vi "OPC Main.vi"(7 "Name of Parent Panel":string="Main.vi", 9 "New Center Coords":T1={"Horizontal"=470, "Vertical"=200}, 10 "Config":variant, 11 "Main UI Message Queue":refnum<queue>) -> ()   [LabVIEW 2018, in "OPC UA.lvlib"]
uses:
  OPC UA.lvlib
  support/Message Queue/Message Cluster.ctl
  <vilib>/Utility/miscctls.llb/LVPoint32TypeDef.ctl
  controls/UI State.ctl
  OPC Module Config.ctl
  Scale Module Folder/Measure Instrument/State Enum.ctl
  OPC Settings.ctl
  Variable Data Cluster.ctl
  <vilib>/OPCUA/controls/NodeId.ctl
  <vilib>/OPCUA/controls/OPC UA StatusCode.ctl
  <vilib>/OPCUA/controls/Subscription ID.ctl
  <vilib>/OPCUA/controls/OPC UA Client Refnum.ctl
  <vilib>/OPCUA/controls/Subscription Data Change.ctl
  <vilib>/OPCUA/controls/Data Type.ctl
  OPC Display Cluster.ctl
  support/Message Queue/Enqueue Message (Single).vi
  <vilib>/Utility/error.llb/Error Cluster From Error Code.vi
  <vilib>/ErrorRing/Error Ring.xnode
  support/Message Queue/Message Queue.lvlib
  support/Support Library.lvlib
  support/Command Log VIs/Command Logging.lvlib
  support/User Event - Stop/User Event - Stop.lvlib
  OPC Dialog.vi
  Scale Module Folder/Measure Instrument/Scale Module Engine.lvlib
  OPC UA Module Engine.lvlib
panel:
  out "Configuration.server endpoint URL":string
  out "Updating":bool
  out "ScanCode":i16
  in  "Settings Button":bool
  in  "Exit":bool
  out "Status":string
  out "Log File path":path
  out "server endpoint URL":string
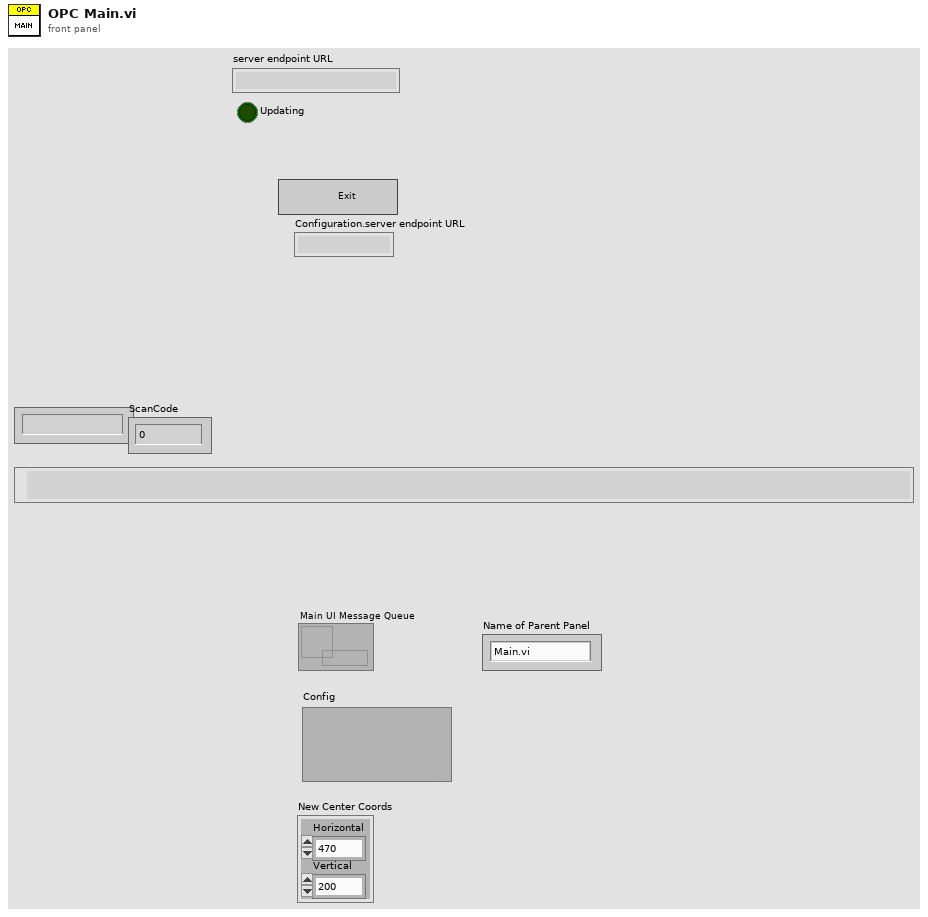
[diagram p1: front panel]
types:
  T1 = typedef "LVPoint32TypeDef.ctl" = cluster{"Horizontal":i32, "Vertical":i32}
  T2 = typedef "OPC UA.lvlib/OPC Module Config.ctl" = cluster{"State":T3, "GUID":string, "Drop Coords":T1, "Configuration":T4, "First Iteration":bool, "Data":cluster{"Object Name":string, "Variable Array":T5[]}[], "Process Name":string, "Load Count":i32, "Log Started":bool, "subscription ID out":T8, "OPC UA client refnum out":T9, "Event Registration Refnum":refnum<event-registration>, "Start Time":timestamp, "Current Time":timestamp}
  T3 = typedef "Scale Module.lvlib/Scale Module Engine.lvlib/State Enum.ctl" = enum16{"Measuring", "Idle"}
  T4 = typedef "OPC UA.lvlib/OPC Settings.ctl" = cluster{"Cycle Period":dbl, "server endpoint URL":string, "security policy":cluster{"message mode":enum16{"None", "Sign", "Sign and Encrypt"}, "security":enum16{"Basic256", "Basic128Rsa15"}}, "Trust Any Server":bool}
  T5 = typedef "OPC UA.lvlib/Variable Data Cluster.ctl" = cluster{"node ID":T6, "browse name":string, "status":T7, "timestamp":timestamp, "value ":variant}
  T6 = typedef "NodeId.ctl" = string
  T7 = typedef "OPC UA StatusCode.ctl" = u32
  T8 = typedef "Subscription ID.ctl" = u32
  T9 = typedef "OPC UA Client Refnum.ctl" = refnum<k21>
  T10 = typedef "UI State.ctl" = enum16{"Idle", "Acquiring and Logging", "Waiting for Exit", "Waiting for Exit (Acq Stopped)", "Waiting for Exit (Log Stopped)", "Waiting for Stop", "Waiting for Stop (Acq Stopped)", "Waiting for Stop (Log Stopped)"}
  T11 = typedef "OPC UA.lvlib/Message Queues.ctl" = cluster{"OPC UI":refnum<queue>, "OPC Engine":refnum<queue>, "OPC Display":refnum<queue>}
  T12 = typedef "OPC UA.lvlib/OPC Display Cluster.ctl" = cluster{"URL":string, "Cycle":i32, "Updating":bool}
  T13 = cluster{"Shift":bool, "Ctrl":bool, "Alt":bool, "Cmd":bool, "Opt":bool}
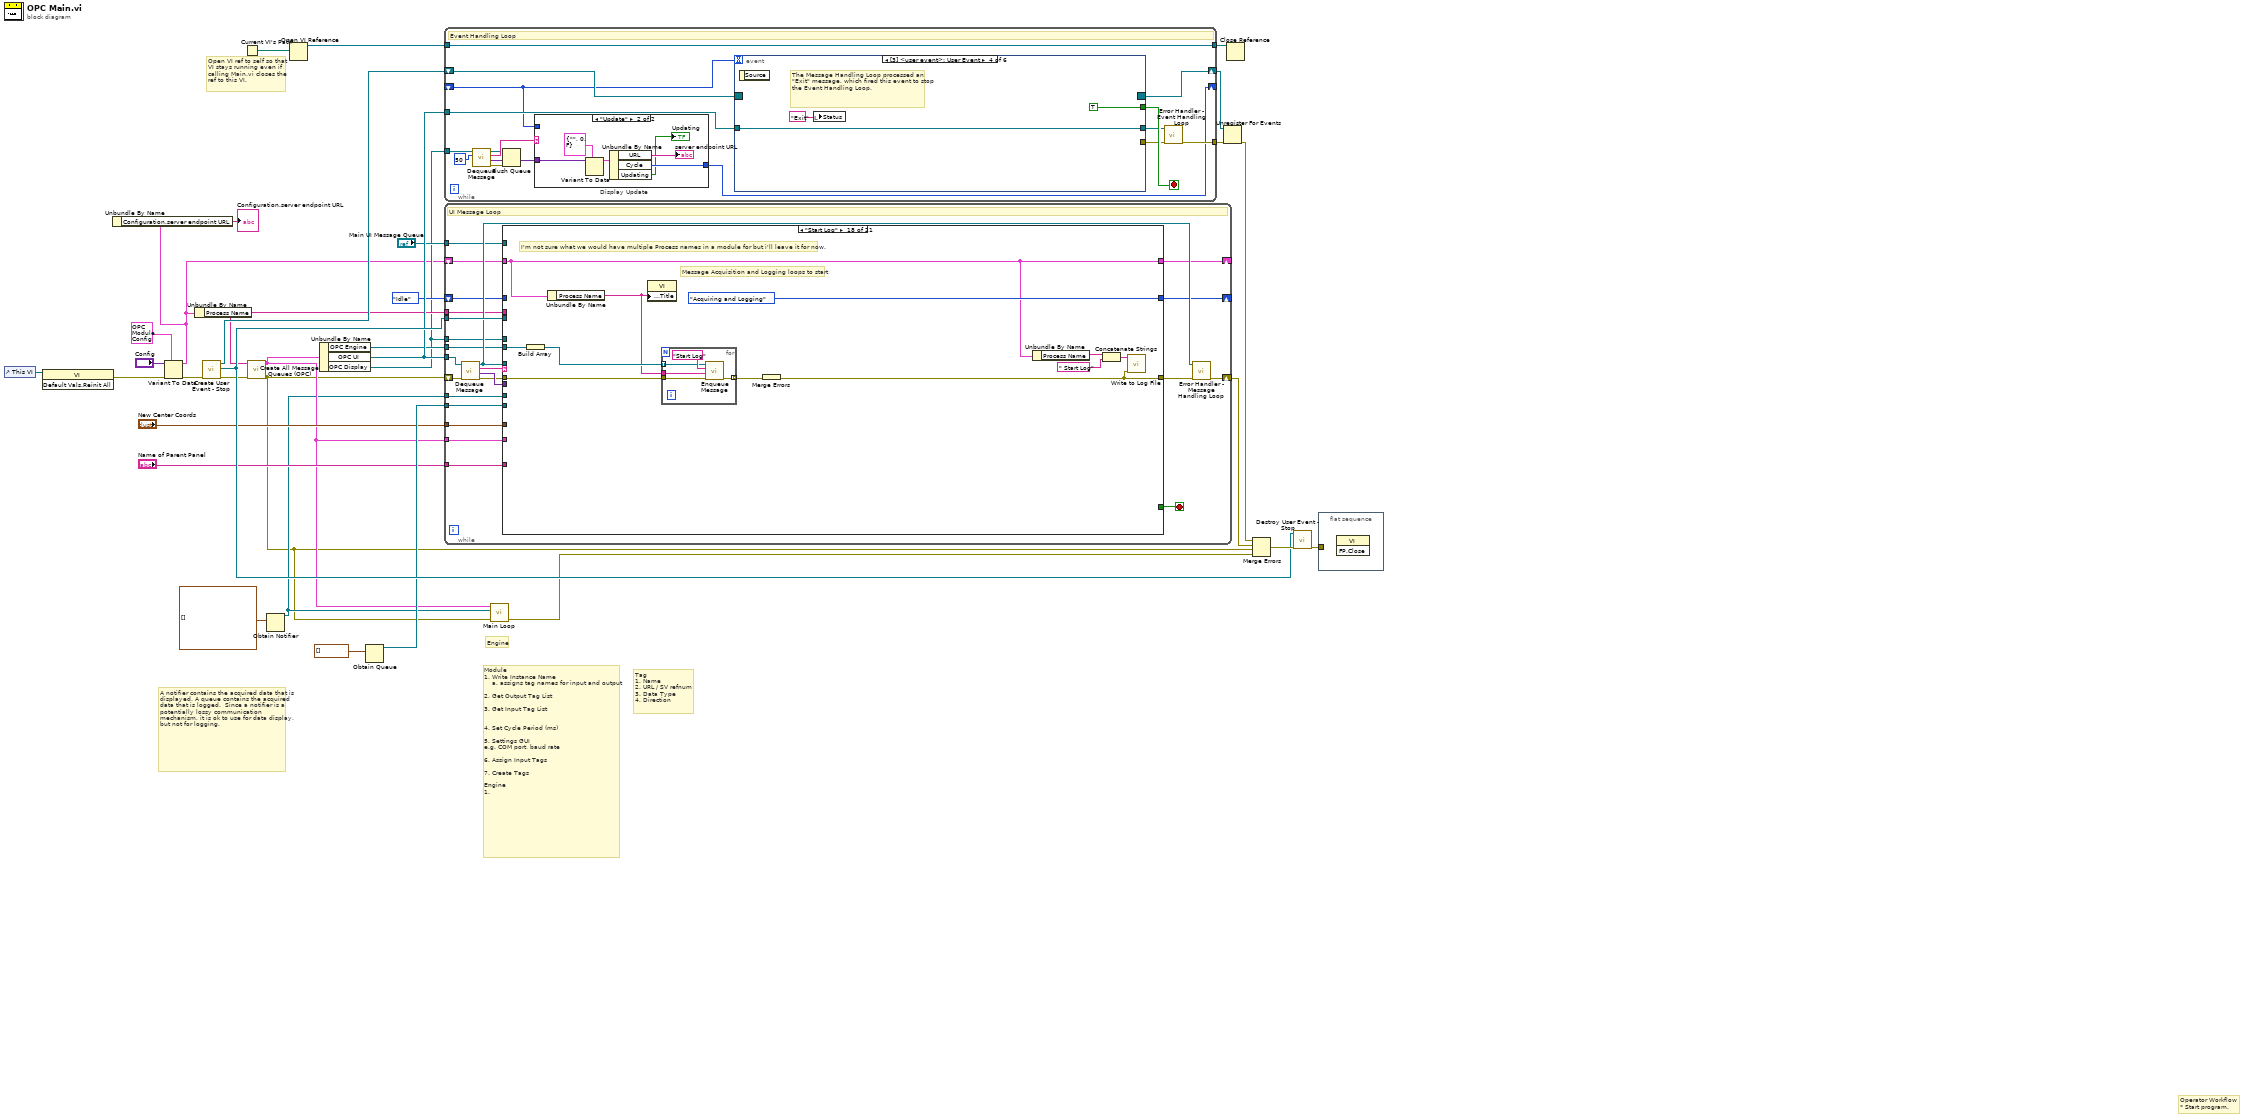
[diagram p0: block diagram]
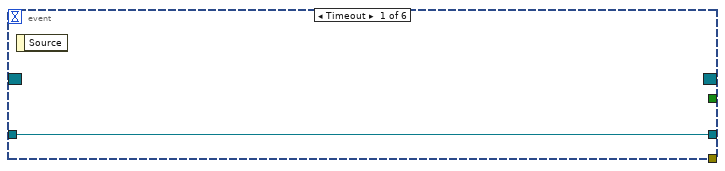
[diagram p3: hidden frame]
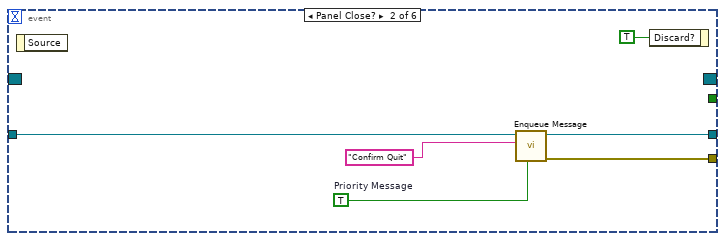
[diagram p4: hidden frame]
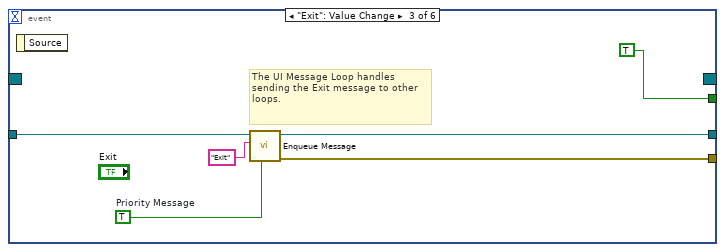
[diagram p5: hidden frame]
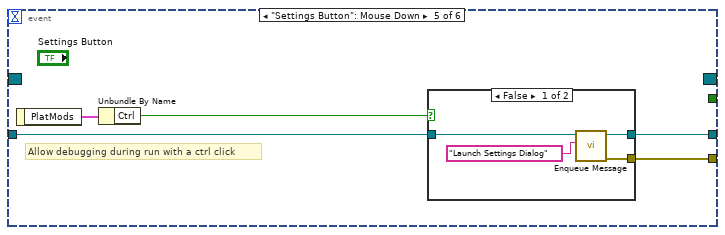
[diagram p6: hidden frame]
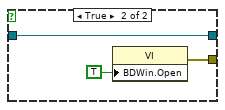
[diagram p7: hidden frame]
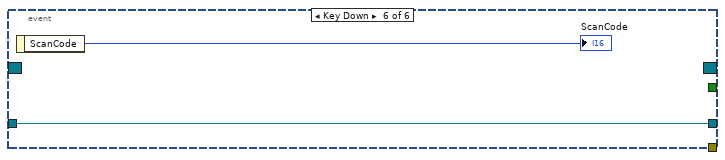
[diagram p8: hidden frame]
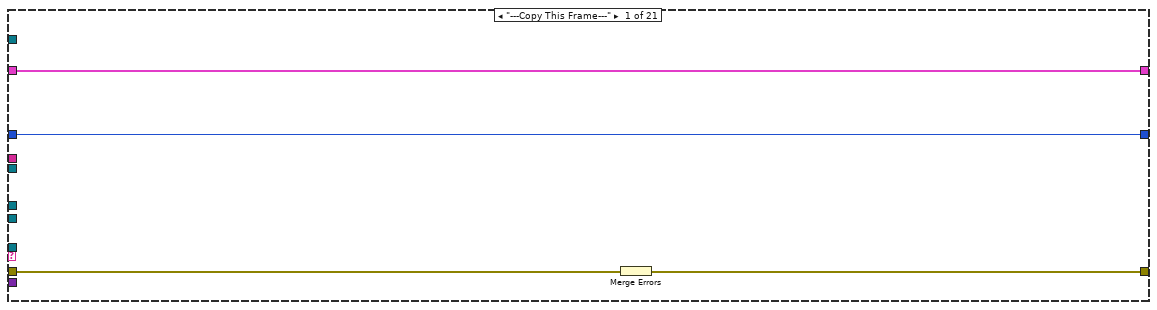
[diagram p9: hidden frame]
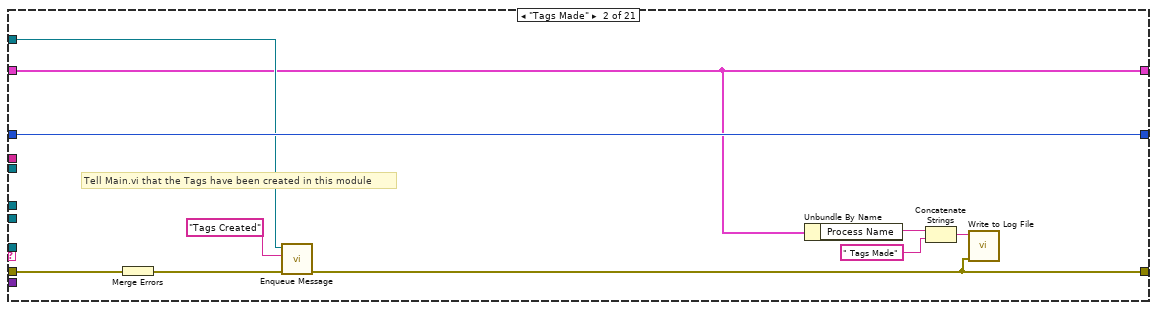
[diagram p10: hidden frame]
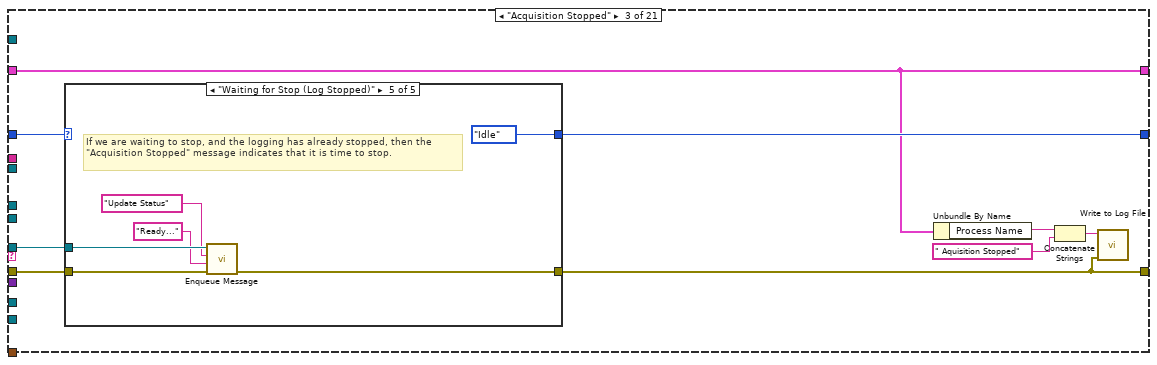
[diagram p11: hidden frame]
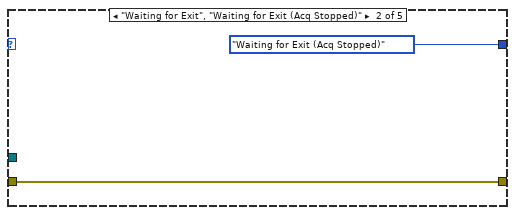
[diagram p13: hidden frame]
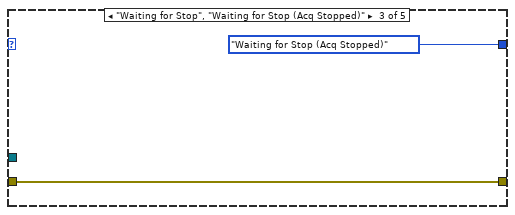
[diagram p14: hidden frame]
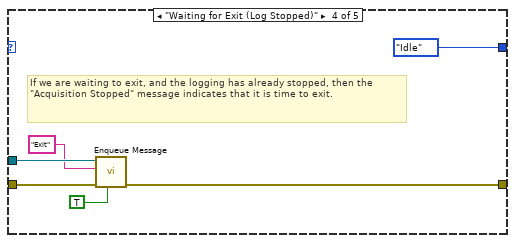
[diagram p15: hidden frame]
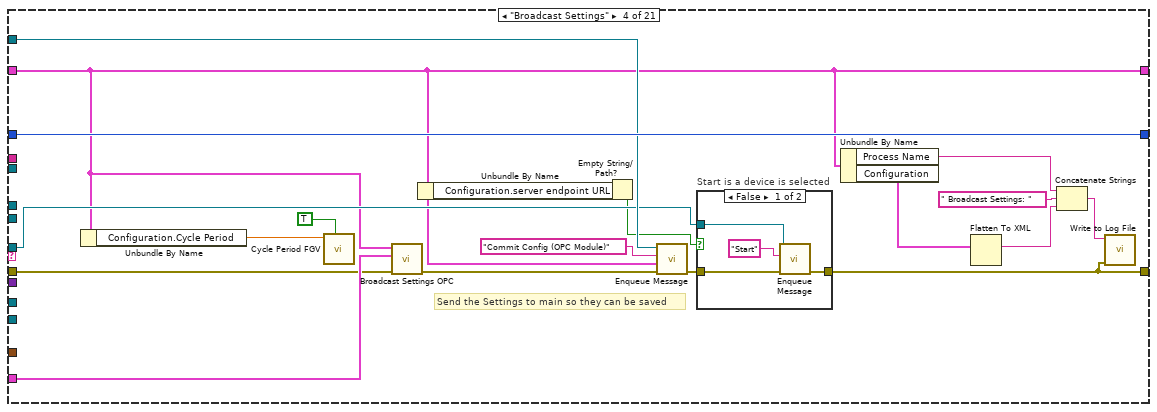
[diagram p16: hidden frame]
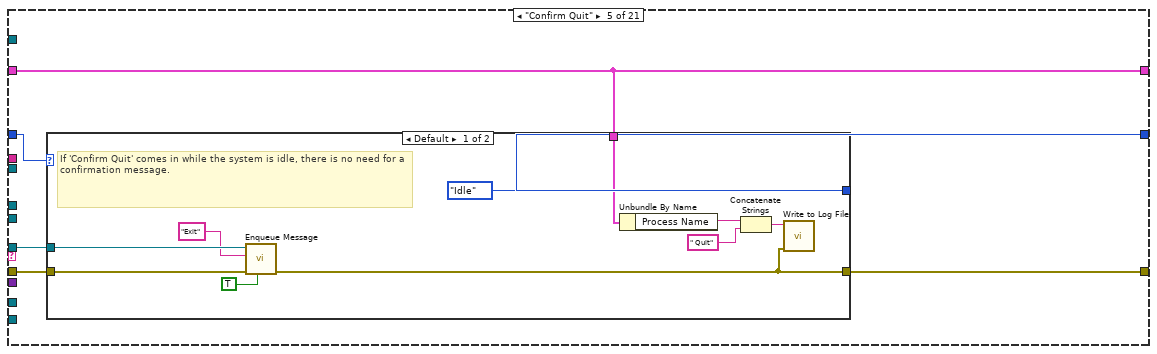
[diagram p18: hidden frame]
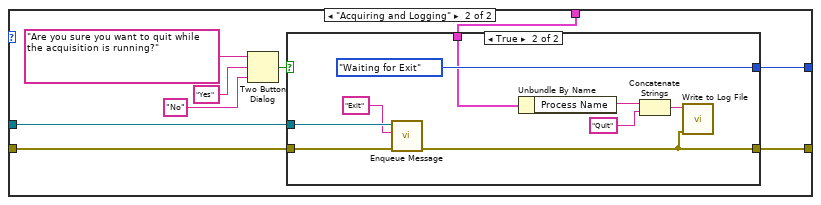
[diagram p19: hidden frame]
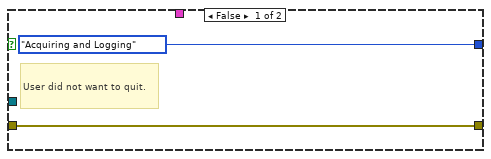
[diagram p20: hidden frame]
diagram:
  # "Open VI ref to self so that\nVI stays running even if\ncalling Main.vi closes the\nref to this VI."
  # "Engine"
  # "Operator Workflow\n* Start program."
  # "Module \n1. Write Instance Name\n    a. assigns tag names for input and output\n\n2. Get Output Tag List\n\n3. Get Input Tag List\n\n\n4. Set Cycle Period (ms)\n\n5. Settings GUI\ne.g. COM port, baud rate\n\n6. Assign Input Tags\n\n7. Create Tags\n\nEngine\n1."
  # "Tag\n1. Name\n2. URL / SV refnum\n3. Data Type\n4. Direction"
  # "A notifier contains the acquired data that is displayed. A queue contains the acquired data that is logged.  Since a notifier is a potentially lossy communication mechanism, it is ok to use for data display, but not for logging."
  n1 = control-ref of="This VI"() -> (w3:refnum<vi>)
  n2 = invoke class="VI" method="Default Vals.Reinit All"(reference=w3) -> (error out=w13:errorcluster)  [unwired: 2 in, 2 out]
  n3 = Variant To Data(error in=w13, type=T2 {"State"=enum."Idle", "GUID"="", "Drop Coords"={"Horizontal"=0, "Vertical"=0}, "Configuration"={"Cycle Period"=500.0, "server endpoint URL"="", "security policy"={"message mode"=enum."Sign", "security"=enum."Basic256"}, "Trust Any Server"=FALSE}, "First Iteration"=FALSE, "Data"=[], "Process Name"="", "Load Count"=0, "Log Started"=FALSE, "subscription ID out"=0, "OPC UA client refnum out"="", "Event Registration Refnum"=refnum, "Start Time"=timestamp(0 s since 1904-01-01), "Current Time"=timestamp(0 s since 1904-01-01)} ("OPC Module Config"), Variant="Config") -> (data=w2:T2, error out=w18:errorcluster)
  n4 = Unbundle By Name(w2) -> ("Configuration.server endpoint URL"=→"Configuration.server endpoint URL":string)
  n5 = Unbundle By Name(w2) -> ("Process Name"=w12:string)
  n6 = call "Create User Event - Stop.vi"("error in (no error)"=w18) -> ("error out"=w11:errorcluster, "User Event - Stop"=w30:refnum<user-event>, "Stop Event Registration Refnum"=w31:refnum<event-registration>)  [unwired: 8 in]
  n7 = Current VI's Path() -> (path=w19:path)
  n8 = call "Create All Message Queues (OPC).vi"("error in (no error)"=w11, "Process Name"=w12) -> ("error out"=w8:errorcluster, "Message Queues"=w10:T11)  [unwired: 8 in]
  n9 = Obtain Notifier(notification data type=waveform(dbl)[] []) -> (notifier out=w9:refnum<notifier>)  [unwired: 3 in, 2 out]
  n10 = Open VI Reference(vi path=w19) -> (vi reference=w20:refnum<vi>)  [unwired: 5 in, 1 out]
  n11 = Unbundle By Name(w10) -> ("OPC Engine"=w23:refnum<queue>, "OPC UI"=w27:refnum<queue>, "OPC Display"=w4:refnum<queue>)
  n12 = Obtain Queue(element data type=waveform(dbl)[] []) -> (queue out=w22:refnum<queue>)  [unwired: 4 in, 2 out]
  n13 = while {
    tunnel: w27 -> [w52]
    tunnel: w30 -> [w56]
    shift-right: [w48] -> w34
    shift-left: w8 -> [w55]
    shift-right: [w39] -> _
    shift-left: w2 -> [w41]
    tunnel: w9 -> [w51]
    tunnel: w22 -> [w50]
    shift-right: [w45] -> _
    shift-left: UI_State."Idle" ("UI State") -> [w46]
    tunnel: w23 -> [w44]
    tunnel: w10 -> [w43]
    tunnel: "Main UI Message Queue" -> [w40]
    tunnel: w12 -> [w38]
    tunnel: "New Center Coords" -> [w37]
    tunnel: "Name of Parent Panel" -> [w36]
    tunnel: w4 -> [w35]
    stop <- w57 stop-if-true
    # "UI Message Loop"
    n14 = call "Dequeue Message.vi"("error in (no error)"=w55, "Message Queue"=w52) -> ("error out"=w42:errorcluster, "Message Data"=w53:variant, "Message"=w54:string, "dup Message Queue"=w47:refnum<queue>)  [unwired: 6 in]
    n15 = case "Message Cases" shown="\"Start Log\"" w54 {
      selector: w54 -> [_ _ _ _ _ _ _ _ _ _ _ _ _ _ _ _ _ _ _ _ w396]
      tunnel: w47 -> [_ _ w77 w112 w127 _ w177 w191 w213 _ w256 w273 w289 w312 w320 w338 _ _ w385 _ _]
      tunnel: w42 -> [w61 w71 w78 w100 w126 w161 w172 w195 w212 w238 w252 w265 w290 w313 w319 w337 w344 w361 w380 w394 _]
      tunnel: [w60 w62 w73 w107 w125 w162 w167 w182 w197 w238 w241 w269 w285 w311 w318 w333 w349 w356 w372 w395 w398] -> w49
      tunnel: [_ _ _ _ _ _ _ _ TRUE _ _ _ _ _ _ _ _ _ _ _ _] -> w57
      tunnel: w53 -> [_ _ _ _ _ w164 _ w194 w202 _ _ _ _ _ _ _ _ _ _ w393 _]
      tunnel: w56 -> [_ _ _ _ _ _ _ _ w223 _ _ _ _ _ _ _ _ _ _ _ _]
      tunnel: w41 -> [w58 w63 w72 w106 w123 w159 w166 w181 w196 w235 w244 w268 w284 w317 w324 w332 w342 w355 w371 w388 w397]
      tunnel: w51 -> [_ _ _ _ _ _ _ _ w221 _ _ _ _ _ _ _ _ _ _ _ _]
      tunnel: w50 -> [_ _ _ _ _ _ _ _ w217 _ _ _ _ _ _ _ _ _ _ _ _]
      tunnel: w46 -> [w59 w70 w80 w117 w128 w160 w173 w186 w210 _ _ w277 w292 w316 w323 _ _ _ w381 w389 w402]
      tunnel: [w59 w70 w79 w117 w124 w160 w174 w186 w209 UI_State."Idle" ("UI State") UI_State."Idle" ("UI State") w277 w291 w316 w323 UI_State."Acquiring and Logging" ("UI State") UI_State."Acquiring and Logging" ("UI State") UI_State."Acquiring and Logging" ("UI State") w382 w389 w402] -> w45
      tunnel: w44 -> [_ _ _ _ _ _ _ _ w216 _ _ _ _ _ _ _ w347 w364 w379 _ _]
      tunnel: w43 -> [_ _ _ w101 _ _ _ _ _ _ _ _ _ _ _ _ _ _ _ _ _]
      tunnel: w40 -> [_ w67 _ w113 _ _ _ _ w201 _ _ w274 _ _ _ _ _ _ _ _ _]
      tunnel: [w58 w63 w72 w106 w123 w159 w166 w181 w196 w235 w244 w263 w284 w317 w324 w332 w342 w355 w371 w388 w397] -> w39
      tunnel: w38 -> [_ _ _ _ _ _ _ _ _ _ w250 _ _ _ _ _ _ _ _ _ _]
      tunnel: w37 -> [_ _ _ _ _ _ _ _ _ _ w249 _ _ _ _ _ _ _ _ _ _]
      tunnel: w36 -> [_ _ _ _ _ _ _ _ _ _ w248 _ _ _ _ _ _ _ _ _ _]
      tunnel: w35 -> [_ _ _ _ _ _ _ _ _ _ w243 _ _ _ _ _ _ _ _ _ _]
      frame "---Copy This Frame---" {
        # "Duplicate this frame when creating new messages.  Change this comment in the duplicated frame to describe this message."
        n16 = Merge Errors(w61) -> (w60:errorcluster)
      }
      frame "Tags Made" {
        # "Tell Main.vi that the Tags have been created in this module"
        # "Duplicate this frame when creating new messages.  Change this comment in the duplicated frame to describe this message."
        n17 = Merge Errors(w71) -> (w68:errorcluster)
        n18 = call-poly "Enqueue Message.vi"("error in (no error)"=w68, "Message"="Tags Created", "Message Queue"=w67) -> ("error out"=w62:errorcluster)  [unwired: 7 in, 1 out]
        n19 = Unbundle By Name(w63) -> ("Process Name"=w66:string)
        n20 = Concatenate Strings(w66, " Tags Made" ("text")) -> (w64:string)
        n21 = call "Write to Log File.vi"("error in"=w62, "text"=w64) -> ()  [unwired: 9 in, 1 out]
      }
      frame "Acquisition Stopped" {
        # "Logic for determining what action to take when the acquisition has stopped."
        n22 = case shown="\"Waiting for Stop (Log Stopped)\"" w80 {
          selector: w80 -> [w82 _ _ _ _]
          tunnel: [w82 UI_State."Waiting for Exit (Acq Stopped)" ("UI State") UI_State."Waiting for Stop (Acq Stopped)" ("UI State") UI_State."Idle" ("UI State") UI_State."Idle" ("UI State")] -> w79
          tunnel: w78 -> [w81 w83 w85 w91 w97]
          tunnel: [w81 w83 w85 w90 w96] -> w73
          tunnel: w77 -> [_ _ _ w89 w95]
          frame Default {
          }
          frame "Waiting for Exit", "Waiting for Exit (Acq Stopped)" {
          }
          frame "Waiting for Stop", "Waiting for Stop (Acq Stopped)" {
          }
          frame "Waiting for Exit (Log Stopped)" {
            # "If we are waiting to exit, and the logging has already stopped, then the \"Acquisition Stopped\" message indicates that it is time to exit."
            n23 = call-poly "Enqueue Message.vi"("Priority Message? (F)"=TRUE, "error in (no error)"=w91, "Message"="Exit", "Message Queue"=w89) -> ("error out"=w90:errorcluster)  [unwired: 6 in, 1 out]
          }
          frame "Waiting for Stop (Log Stopped)" {
            # "If we are waiting to stop, and the logging has already stopped, then the \"Acquisition Stopped\" message indicates that it is time to stop."
            n24 = call-poly "Enqueue Message.vi"("error in (no error)"=w97, "Message Data"="Ready..." ("Message"), "Message"="Update Status", "Message Queue"=w95) -> ("error out"=w96:errorcluster)  [unwired: 6 in, 1 out]
          }
        }
        n25 = Unbundle By Name(w72) -> ("Process Name"=w76:string)
        n26 = Concatenate Strings(w76, " Aquisition Stopped" ("text")) -> (w74:string)
        n27 = call "Write to Log File.vi"("error in"=w73, "text"=w74) -> ()  [unwired: 9 in, 1 out]
      }
      frame "Broadcast Settings" {
        # "Send the Settings to main so they can be saved"
        # "Send the 'Update Settings' message to the Logging and Acquisition message loops."
        n28 = Unbundle By Name(w106) -> ("Configuration.Cycle Period"=w115:dbl)
        n29 = call "Cycle Period FGV.vi"("Write"=TRUE, "Cycle Period In (ms)"=w115) -> ()  [unwired: 8 in, 2 out]
        n30 = call "Broadcast Settings OPC.vi"("error in (no error)"=w100, "Message Queues"=w101, "OPC Module Config"=w106) -> ("error out"=w99:errorcluster)  [unwired: 8 in]
        n31 = Unbundle By Name(w106) -> ("Configuration.server endpoint URL"=w103:string)
        n32 = Empty String/Path?(string/path=w103) -> (empty?=w102:bool)
        n33 = call-poly "Enqueue Message.vi"("error in (no error)"=w99, "Message Data"=w106, "Message"="Commit Config (OPC Module)", "Message Queue"=w113) -> ("error out"=w111:errorcluster)  [unwired: 6 in, 1 out]
        n34 = case "Start is a device is selected" shown="False" w102 {
          tunnel: w112 -> [w120 _]
          tunnel: w111 -> [w119 w122]
          tunnel: [w118 w122] -> w107
          frame False {
            n35 = call-poly "Enqueue Message.vi"("error in (no error)"=w119, "Message"="Start", "Message Queue"=w120) -> ("error out"=w118:errorcluster)  [unwired: 7 in, 1 out]
          }
          frame True {
          }
        }
        n36 = Unbundle By Name(w106) -> ("Process Name"=w110:string, "Configuration"=w105:T4)
        n37 = Flatten To XML(anything=w105) -> (xml string=w104:string)
        n38 = Concatenate Strings(w110, " Broadcast Settings: " ("text"), w104) -> (w108:string)
        n39 = call "Write to Log File.vi"("error in"=w107, "text"=w108) -> ()  [unwired: 9 in, 1 out]
      }
      frame "Confirm Quit" {
        # "Confirm Quit - Message that can confirm whether or not the user wants to exit the application."
        n40 = case shown="Default" w128 {
          tunnel: w127 -> [w137 w144]
          tunnel: w126 -> [w136 w142]
          tunnel: [w130 w141] -> w125
          tunnel: [UI_State."Idle" ("UI State") w140] -> w124
          tunnel: w123 -> [w129 w139]
          frame Default {
            # "If 'Confirm Quit' comes in while the system is idle, there is no need for a confirmation message."
            n41 = call-poly "Enqueue Message.vi"("Priority Message? (F)"=TRUE, "error in (no error)"=w136, "Message"="Exit", "Message Queue"=w137) -> ("error out"=w130:errorcluster)  [unwired: 6 in, 1 out]
            n42 = Unbundle By Name(w129) -> ("Process Name"=w133:string)
            n43 = Concatenate Strings(w133, " Quit" ("text")) -> (w131:string)
            n44 = call "Write to Log File.vi"("error in"=w130, "text"=w131) -> ()  [unwired: 9 in, 1 out]
          }
          frame "Acquiring and Logging" {
            n45 = Two Button Dialog(message="Are you sure you want to quit while the acquisition is running?" ("Confirm Quit Message"), 1:"No" ("No"), 2:"Yes" ("Yes")) -> (T button?=w143:bool)
            n46 = case shown="True" w143 {
              tunnel: w144 -> [_ w158]
              tunnel: w142 -> [w148 w157]
              tunnel: [w148 w151] -> w141
              tunnel: [UI_State."Acquiring and Logging" ("UI State") UI_State."Waiting for Exit" ("UI State")] -> w140
              tunnel: w139 -> [_ w150]
              frame False {
                # "User did not want to quit."
              }
              frame True {
                n47 = call-poly "Enqueue Message.vi"("error in (no error)"=w157, "Message"="Exit", "Message Queue"=w158) -> ("error out"=w151:errorcluster)  [unwired: 7 in, 1 out]
                n48 = Unbundle By Name(w150) -> ("Process Name"=w154:string)
                n49 = Concatenate Strings(w154, "Quit" ("text")) -> (w152:string)
                n50 = call "Write to Log File.vi"("error in"=w151, "text"=w152) -> ()  [unwired: 9 in, 1 out]
              }
            }
          }
        }
      }
      frame "Display Log File Path" {
        n51 = Variant To Data(error in=w161, type=path "", Variant=w164) -> (data=→"Log File path":path, error out=w162:errorcluster)
      }
      frame "E-Stop" {
        # "E-Stop has no effect on the scale"
        # "Message Acquisition and Logging loops to stop"
        # "Stop the pumps."
        n52 = call-poly "Enqueue Message.vi"("error in (no error)"=w172, "Message Data"="Ready..." ("Ready..."), "Message"="Update Status", "Message Queue"=w177) -> ("error out"=w171:errorcluster)  [unwired: 6 in, 1 out]
        n53 = case shown="\"Waiting for Exit\"" w173 {
          selector: w173 -> [_ w179]
          tunnel: [UI_State."Waiting for Stop" ("UI State") w179] -> w174
          frame Default {
          }
          frame "Waiting for Exit" {
          }
        }
        n54 = Merge Errors(w171) -> (w167:errorcluster)
        n55 = Unbundle By Name(w166) -> ("Process Name"=w170:string)
        n56 = Concatenate Strings(w170, " E-STOP" ("text")) -> (w168:string)
        n57 = call "Write to Log File.vi"("error in"=w167, "text"=w168) -> ()  [unwired: 9 in, 1 out]
      }
      frame "Error" {
        # "Error - Check the error message data and respond accordingly. This message is sent by the \"Error Handler\" VIs at the end of each loop in this application."
        n58 = Variant To Data(error in=w195, type=errorcluster {"status"=FALSE, "code"=0, "source"=""} ("error out"), Variant=w194) -> (data=w192:errorcluster, error out=w188:errorcluster)
        n59 = call <vilib>:"General Error Handler.vi"("error in (no error)"=w192) -> ("message"=w180:string)  [unwired: 10 in, 4 out]
        n60 = call-poly "Enqueue Message.vi"("Priority Message? (F)"=TRUE, "Message"="Exit", "Message Queue"=w191) -> ("error out"=w187:errorcluster)  [unwired: 7 in, 1 out]
        n61 = Merge Errors(w187, w188) -> (w182:errorcluster)
        n62 = Unbundle By Name(w181) -> ("Process Name"=w185:string)
        n63 = Concatenate Strings(w185, " Error: " ("text"), w180) -> (w183:string)
        n64 = call "Write to Log File.vi"("error in"=w182, "text"=w183) -> ()  [unwired: 9 in, 1 out]
      }
      frame "Exit" {
        w205 = TRUE  # Delete Module?
        # "Don't check the error outs. The acquisition and logging queues may have already been released."
        # "Close references owned by the Main VI."
        # "Stop the VI"
        # "Exit - Fire the User Event to stop the Event Handling Loop.  Also send Exit messages to the Acquisition and Logging loops."
        n65 = call "Fire User Event - Stop.vi"("User Event - Stop"=w223) -> ("error out"=w222:errorcluster)  [unwired: 10 in]
        n66 = Build Array(w216) -> (w215:refnum<queue>[])
        n67 = for {
          tunnel: w215 -> [w232] mode=indexing
          n68 = call-poly "Enqueue Message.vi"("Message"="Stop", "Message Queue"=w232) -> ("dup Message Queue"=w233:refnum<queue>)  [unwired: 8 in, 1 out]
          n69 = call-poly "Enqueue Message.vi"("Message"="Exit", "Message Queue"=w233) -> ()  [unwired: 8 in, 2 out]
        }
        n70 = Variant To Data(type=w205, Variant=w202) -> (data=w204:bool, error out=w206:errorcluster)  [unwired: 1 in]
        n71 = call-poly "Enqueue Message.vi"("error in (no error)"=w212, "Message Data"="Ready..." ("Ready..."), "Message"="Update Status", "Message Queue"=w213) -> ("error out"=w211:errorcluster, "dup Message Queue"=w208:refnum<queue>)  [unwired: 6 in]
        n72 = Select(t=w205, s=w206, f=w204) -> (s? t:f=w203:bool)
        n73 = case "Don't enqueue Delete Module if opening campaign because it\nwill already have been deleted and new config loaded and we create\na race condition." shown="True" w203 {
          tunnel: w201 -> [_ w227]
          tunnel: w196 -> [_ w226]
          frame False {
          }
          frame True {
            n74 = Unbundle By Name(w226) -> ("GUID"=w225:string)
            n75 = call-poly "Enqueue Message.vi"("Message Data"=w225, "Message"="Delete Module", "Message Queue"=w227) -> ()  [unwired: 7 in, 2 out]
          }
        }
        n76 = Release Queue(queue=w208, error in (no error)=w211) -> (error out=w220:errorcluster)  [unwired: 1 in, 2 out]
        n77 = Release Notifier(notifier=w221, error in (no error)=w220) -> (error out=w219:errorcluster)  [unwired: 1 in, 2 out]
        n78 = Release Queue(queue=w217, error in (no error)=w219) -> (error out=w218:errorcluster)  [unwired: 1 in, 2 out]
        n79 = Merge Errors(w222, w218) -> (w197:errorcluster)
        n80 = case shown="Default" w210 {
          selector: w210 -> [_ w230]
          tunnel: [UI_State."Waiting for Stop" ("UI State") w230] -> w209
          frame Default {
          }
          frame "Waiting for Exit" {
          }
        }
        n81 = Unbundle By Name(w196) -> ("Process Name"=w200:string)
        n82 = Concatenate Strings(w200, " Exit" ("text")) -> (w198:string)
        n83 = call "Write to Log File.vi"("error in"=w197, "text"=w198) -> ()  [unwired: 9 in, 1 out]
      }
      frame "Init UI Refs" {
        # "Init UI Refs - Store control references for UI controls.  Also enable/disable controls appropriately."
        n84 = property class="VI"("Front Panel.Closeable"=TRUE ("Front Panel Window:Closeable")) -> ()  [unwired: 2 in, 2 out]
      }
      frame "Initialize" {
        # "Initialize - Get configuration settings, then message the UI to initialize, and broadcast the settings to the other message loops."
        n85 = call-poly "Enqueue Message.vi"("error in (no error)"=w252, "Message"="Init UI Refs", "Message Queue"=w256) -> ("error out"=w254:errorcluster, "dup Message Queue"=w255:refnum<queue>)  [unwired: 7 in]
        n86 = property class="VI" props=["FP.State"]() -> (reference out=w251:refnum<vi>)  [unwired: 2 in, 2 out]
        n87 = call "Make Child and Move.vi"("Process Name"=w250, "Name of Parent Panel"=w248, "New Center Coords"=w249, "VI in"=w251) -> ()  [unwired: 8 in]
        n88 = call-poly "Enqueue Message.vi"("error in (no error)"=w254, "Message"="Broadcast Settings", "Message Queue"=w255) -> ("error out"=w262:errorcluster, "dup Message Queue"=w261:refnum<queue>)  [unwired: 7 in]
        n89 = call-poly "Enqueue Message.vi"("error in (no error)"=w262, "Message Data"="Ready..." ("Ready..."), "Message"="Update Status", "Message Queue"=w261) -> ("error out"=w242:errorcluster)  [unwired: 6 in, 1 out]
        n90 = call-poly "Enqueue Message.vi"("error in (no error)"=w242, "Message Data"=T12 {"URL"="", "Cycle"=0, "Updating"=FALSE} ("OPC Display Cluster"), "Message"="Update", "Message Queue"=w243) -> ("error out"=w241:errorcluster)  [unwired: 6 in, 1 out]
        n91 = Unbundle By Name(w244) -> ("Process Name"=w247:string)
        n92 = Concatenate Strings(w247, " Initialize" ("text")) -> (w245:string)
        n93 = call "Write to Log File.vi"("error in"=w241, "text"=w245) -> ()  [unwired: 9 in, 1 out]
      }
      frame "Launch Settings Dialog" {
        # "Launch the Settings Dialog when the user clicks the 'Settings' button."
        n94 = Unbundle By Name(w268) -> ("Load Count"=w275:i32)
        n95 = Increment(x=w275) -> (x+1=w276:i32)
        n96 = Bundle By Name(cluster=w268, "Load Count"=w276) -> (w264:T2)
        n97 = call-by-ref "?"("error in (no error)"=w265, "OPC Module Config In"=w264) -> ("error out"=w266:errorcluster, "Cancelled?"=w267:bool, "OPC Module Config Out"=w263:T2)  [unwired: 8 in, 3 out]
        n98 = case shown="False" w267 {
          tunnel: w266 -> [w280 w283]
          tunnel: [w279 w283] -> w269
          tunnel: w274 -> [_ _]
          tunnel: w273 -> [w282 _]
          tunnel: w263 -> [w278 _]
          frame False {
            n99 = call-poly "Enqueue Message.vi"("error in (no error)"=w280, "Message Data"=w278, "Message"="Broadcast Settings", "Message Queue"=w282) -> ("error out"=w279:errorcluster)  [unwired: 6 in, 1 out]
          }
          frame True {
          }
        }
        n100 = Unbundle By Name(w263) -> ("Process Name"=w272:string)
        n101 = Concatenate Strings(w272, " Setting Dialog Launched" ("text")) -> (w270:string)
        n102 = call "Write to Log File.vi"("error in"=w269, "text"=w270) -> ()  [unwired: 9 in, 1 out]
      }
      frame "Logging Stopped" {
        # "Logic for determining what action to take when the logging has stopped."
        n103 = case shown="\"Waiting for Exit (Acq Stopped)\"" w292 {
          selector: w292 -> [w294 _ _ _ _]
          tunnel: [w294 UI_State."Waiting for Exit (Log Stopped)" ("UI State") UI_State."Waiting for Stop (Log Stopped)" ("UI State") UI_State."Idle" ("UI State") UI_State."Idle" ("UI State")] -> w291
          tunnel: w290 -> [w293 w295 w297 w303 w309]
          tunnel: [w293 w295 w297 w302 w308] -> w285
          tunnel: w289 -> [_ _ _ w301 w307]
          frame Default {
          }
          frame "Waiting for Exit", "Waiting for Exit (Log Stopped)" {
          }
          frame "Waiting for Stop", "Waiting for Stop (Log Stopped)" {
          }
          frame "Waiting for Exit (Acq Stopped)" {
            # "If we are waiting to exit, and the acquisition has already stopped, then the \"Logging Stopped\" message indicates that it is time to exit."
            n104 = call-poly "Enqueue Message.vi"("Priority Message? (F)"=TRUE, "error in (no error)"=w303, "Message"="Exit", "Message Queue"=w301) -> ("error out"=w302:errorcluster)  [unwired: 6 in, 1 out]
          }
          frame "Waiting for Stop (Acq Stopped)" {
            # "If we are waiting to stop, and the acquisition has already stopped, then the \"Logging Stopped\" message indicates that it is time to stop."
            n105 = call-poly "Enqueue Message.vi"("error in (no error)"=w309, "Message Data"="Ready..." ("Message"), "Message"="Update Status", "Message Queue"=w307) -> ("error out"=w308:errorcluster)  [unwired: 6 in, 1 out]
          }
        }
        n106 = Unbundle By Name(w284) -> ("Process Name"=w288:string)
        n107 = Concatenate Strings(w288, " Logging Stopped" ("text")) -> (w286:string)
        n108 = call "Write to Log File.vi"("error in"=w285, "text"=w286) -> ()  [unwired: 9 in, 1 out]
      }
      frame "Send to Sequencer" {
        n109 = local read "Status"() -> (w314:string)
        n110 = call-poly "Enqueue Message.vi"("error in (no error)"=w313, "Message Data"=w314, "Message"="Sent to Sequence", "Message Queue"=w312) -> ("error out"=w311:errorcluster)  [unwired: 6 in, 1 out]
      }
      frame "Sent to Sequence" {
        n111 = local read "Status"() -> (w321:string)
        n112 = flat-sequence {
          tunnel: w319 -> [w329]
          tunnel: w320 -> [w327]
          tunnel: [w328] -> w322
          tunnel: w321 -> [w325]
          tunnel: [w331] -> w318
          tunnel: w322 -> [w331]
          frame #0 {
            n113 = call-poly "Enqueue Message.vi"("error in (no error)"=w329, "Message Data"=w325, "Message"="Sent to Sequence", "Message Queue"=w327) -> ("error out"=w328:errorcluster)  [unwired: 6 in, 1 out]
          }
          frame #1 {
            n114 = Wait (ms)(milliseconds to wait=u32 50) -> ()  [unwired: 1 out]
          }
        }
      }
      frame "Start" {
        # "Message Acquisition and Logging loops to start"
        # "Start - Enable/Disable buttons appropriately for an acquisition that has started, and update status display."
        n115 = call-poly "Enqueue Message.vi"("error in (no error)"=w337, "Message"="Start Loops", "Message Queue"=w338) -> ("error out"=w339:errorcluster)  [unwired: 7 in, 1 out]
        n116 = Merge Errors(w339) -> (w333:errorcluster)
        n117 = Unbundle By Name(w332) -> ("Process Name"=w336:string)
        n118 = Concatenate Strings(w336, " Start" ("text")) -> (w334:string)
        n119 = call "Write to Log File.vi"("error in"=w333, "text"=w334) -> ()  [unwired: 9 in, 1 out]
      }
      frame "Start Loops" {
        # "I'm not sure what we would have multiple Process names in a module for but i'll leave it for now."
        # "Message Acquisition and Logging loops to start"
        # "Start - Enable/Disable buttons appropriately for an acquisition that has started, and update status display."
        n120 = Build Array(w347) -> (w345:refnum<queue>[])
        n121 = Unbundle By Name(w342) -> ("Process Name"=w343:string)
        n122 = property class="VI"("Front Panel.Title"=w343) -> ()  [unwired: 2 in, 2 out]
        n123 = for {
          tunnel: w344 -> [w353]
          tunnel: [w352] -> w346 mode=indexing
          tunnel: w345 -> [w351] mode=indexing
          tunnel: w343 -> [w350]
          n124 = call-poly "Enqueue Message.vi"("error in (no error)"=w353, "Message Data"=w350, "Message"="Start", "Message Queue"=w351) -> ("error out"=w352:errorcluster)  [unwired: 6 in, 1 out]
        }
        n125 = Merge Errors(w346) -> (w349:errorcluster)
      }
      frame "Start Log" {
        # "I'm not sure what we would have multiple Process names in a module for but i'll leave it for now."
        # "Message Acquisition and Logging loops to start"
        # "Start - Enable/Disable buttons appropriately for an acquisition that has started, and update status display."
        n126 = Build Array(w364) -> (w362:refnum<queue>[])
        n127 = Unbundle By Name(w355) -> ("Process Name"=w360:string)
        n128 = property class="VI"("Front Panel.Title"=w360) -> ()  [unwired: 2 in, 2 out]
        n129 = for {
          tunnel: w361 -> [w369]
          tunnel: [w368] -> w363 mode=indexing
          tunnel: w362 -> [w367] mode=indexing
          tunnel: w360 -> [w366]
          n130 = call-poly "Enqueue Message.vi"("error in (no error)"=w369, "Message Data"=w366, "Message"="Start Log", "Message Queue"=w367) -> ("error out"=w368:errorcluster)  [unwired: 6 in, 1 out]
        }
        n131 = Merge Errors(w363) -> (w356:errorcluster)
        n132 = Unbundle By Name(w355) -> ("Process Name"=w359:string)
        n133 = Concatenate Strings(w359, " Start Log" ("text")) -> (w357:string)
        n134 = call "Write to Log File.vi"("error in"=w356, "text"=w357) -> ()  [unwired: 9 in, 1 out]
      }
      frame "Stop" {
        # "Stop - Enable/Disable buttons appropriately for an acquisition that has stopped, and update status display."
        n135 = call-poly "Enqueue Message.vi"("error in (no error)"=w380, "Message Data"="Ready..." ("Ready..."), "Message"="Update Status", "Message Queue"=w385) -> ("error out"=w378:errorcluster)  [unwired: 6 in, 1 out]
        n136 = call-poly "Enqueue Message.vi"("error in (no error)"=w378, "Message"="Stop", "Message Queue"=w379) -> ("error out"=w376:errorcluster)  [unwired: 7 in, 1 out]
        n137 = case shown="Default" w381 {
          selector: w381 -> [_ w387]
          tunnel: [UI_State."Waiting for Stop" ("UI State") w387] -> w382
          frame Default {
          }
          frame "Waiting for Exit" {
          }
        }
        n138 = Merge Errors(w376) -> (w372:errorcluster)
        n139 = Unbundle By Name(w371) -> ("Process Name"=w375:string)
        n140 = Concatenate Strings(w375, " Stop" ("text")) -> (w373:string)
        n141 = call "Write to Log File.vi"("error in"=w372, "text"=w373) -> ()  [unwired: 9 in, 1 out]
      }
      frame "Update Status" {
        # "Update Display - Convert the message data to a string to display in the Status indicator."
        n142 = Variant To Data(error in=w394, type="", Variant=w393) -> (data=→"Status":string, error out=w391:errorcluster)
        n143 = Merge Errors(w391) -> (w395:errorcluster)
      }
      frame Default {
        # "'Default' case only runs if there is a message that isn't defined in any of the other cases.  Output a programming error."
        n144 = xnode "Error Ring"("parameter 0"=w396) -> ("error out"=w398:errorcluster)
        n145 = Unbundle By Name(w397) -> ("Process Name"=w401:string)
        n146 = Concatenate Strings(w401, "Invalid Message Recieved" ("text"), w396) -> (w399:string)
        n147 = call "Write to Log File.vi"("error in"=w398, "text"=w399) -> ()  [unwired: 9 in, 1 out]
      }
    }
    n148 = call "Error Handler - Message Handling Loop.vi"("error in (no error)"=w49, "Message Queue"=w47) -> ("dup error in"=w48:errorcluster)  [unwired: 8 in, 1 out]
  }
  n149 = while {
    tunnel: w27 -> [w419]
    tunnel: [w421] -> w33
    shift-right: [w420] -> w28
    shift-left: w31 -> [w425]
    tunnel: [w418] -> w21
    tunnel: w20 -> [w418]
    tunnel: w4 -> [w417]
    shift-right: [w410] -> _
    shift-left: _ -> [w411]
    stop <- w424 stop-if-true
    # "Event Handling Loop"
    n150 = call "Dequeue Message.vi"("timeout in ms (-1)"=50, "Message Queue"=w417) -> ("error out"=w412:errorcluster, "Message Data"=w415:variant, "Message"=w416:string, "dup Message Queue"=w413:refnum<queue>)  [unwired: 6 in]
    n151 = Flush Queue(queue=w413, error in (no error)=w412) -> ()  [unwired: 3 out]
    n152 = case "Display Update" shown="\"Update\"" w416 {
      tunnel: w415 -> [_ w432]
      tunnel: w411 -> [w426 _]
      tunnel: [w426 w429] -> w410
      frame "False", Default {
      }
      frame "Update" {
        n153 = Variant To Data(type=T12 {"URL"="", "Cycle"=0, "Updating"=FALSE} ("OPC Display Cluster"), Variant=w432) -> (data=w431:T12)  [unwired: 1 in, 1 out]
        n154 = Unbundle By Name(w431) -> ("URL"=→"server endpoint URL":string, "Cycle"=w429:i32, "Updating"=→"Updating":bool)
      }
    }
    n155 = event shown="[3] <user event>: User Event" {
      selector: w425 -> [_ _ _ _ _ _]
      dyn-events: [_ _ _ _ _ _] -> w420
      timeout: w411 -> [_ _ _ _ _ _]
      tunnel: [_ _ TRUE ("Discard?") TRUE ("Discard?") _ _] -> w424
      tunnel: w419 -> [w433 w436 w440 w446 w451 w461]
      tunnel: [_ w434 w445 _ w453 _] -> w422
      tunnel: [w433 w435 w443 w446 w452 w461] -> w423
      event Timeout {
        n156 = event-data() -> ()  [unwired: 1 in, 1 out]
      }
      event Panel Close? {
        w437 = TRUE  # Priority Message
        n157 = event-data() -> ()  [unwired: 1 in, 1 out]
        n158 = call-poly "Enqueue Message.vi"("Priority Message? (F)"=w437, "Message"="Confirm Quit", "Message Queue"=w436) -> ("error out"=w434:errorcluster, "dup Message Queue"=w435:refnum<queue>)  [unwired: 7 in]
        n159 = event-data("Discard?"=TRUE) -> ()  [unwired: 1 in, 1 out]
      }
      event "Exit": Value Change {
        w441 = TRUE  # Priority Message
        # "The UI Message Loop handles sending the Exit message to other loops."
        n160 = event-data() -> ()  [unwired: 1 in, 1 out]
        n161 = call-poly "Enqueue Message.vi"("Priority Message? (F)"=w441, "Message"="Exit", "Message Queue"=w440) -> ("error out"=w445:errorcluster, "dup Message Queue"=w443:refnum<queue>)  [unwired: 7 in]
      }
      event User Event {
        # "The Message Handling Loop processed an \"Exit\" message, which fired this event to stop the Event Handling Loop."
        n162 = event-data() -> ()  [unwired: 1 in, 1 out]
        n163 = local write "Status"("Exit" ("Exit String")) -> ()
      }
      event "Settings Button": Mouse Down {
        # "Allow debugging during run with a ctrl click"
        n164 = event-data() -> ("PlatMods"=w450:T13)  [unwired: 1 in]
        n165 = Unbundle By Name(w450) -> ("Ctrl"=w449:bool)
        n166 = case shown="False" w449 {
          tunnel: [w457 w458] -> w453
          tunnel: [w456 w459] -> w452
          tunnel: w451 -> [w455 w459]
          frame False {
            n167 = call-poly "Enqueue Message.vi"("Message"="Launch Settings Dialog", "Message Queue"=w455) -> ("error out"=w457:errorcluster, "dup Message Queue"=w456:refnum<queue>)  [unwired: 8 in]
          }
          frame True {
            n168 = property class="VI"("BDWin.Open"=TRUE ("Block Diagram Window:Open")) -> (error out=w458:errorcluster)  [unwired: 2 in, 1 out]
          }
        }
      }
      event Key Down {
        n169 = event-data() -> ("ScanCode"=→"ScanCode":i16)  [unwired: 1 in]
      }
    }
    n170 = call "Error Handler - Event Handling Loop.vi"("error in (no error)"=w422, "Message Queue"=w423) -> ("dup error in"=w421:errorcluster)  [unwired: 8 in, 1 out]
  }
  n171 = call "Main Loop.vi"("error in (no error)"=w8, "Chart Notifier"=w9, "Message Queues"=w10) -> ("error out"=w7:errorcluster)  [unwired: 8 in]
  n172 = Unregister For Events(event registration refnum=w28, error in=w33) -> (error out=w29:errorcluster)
  n173 = Close Reference(reference=w21) -> ()  [unwired: 1 in, 1 out]
  n174 = Merge Errors(w29, w34, w8, w7) -> (w32:errorcluster)
  n175 = call "Destroy User Event - Stop.vi"("error in (no error)"=w32, "User Event - Stop"=w30) -> ("error out"=w14:errorcluster)  [unwired: 9 in]
  n176 = flat-sequence {
    tunnel: w14 -> [_]
    frame #0 {
      n177 = invoke class="VI" method="FP.Close"() -> ()  [unwired: 3 in, 3 out]
    }
  }
